vi "UpdateUserInterface.vi"(8 "error in (no error)":errorcluster, 10 "DataExchange":T1, 11 "LaserController in":refnum<class "LaserController.lvclass">) -> (0 "error out":errorcluster, 2 "DataExchange Out":T1, 3 "LaserController out":refnum<class "LaserController.lvclass">)   [LabVIEW 2020, in "LaserController.lvlib" / "LaserController.lvclass"]
uses:
  LaserController.lvclass
  Model/Hardware Abstraction Layer/Component/Device/Device/DataExchange.ctl
  LaserController.lvclass/LaserController.ctl
  Model/Hardware Abstraction Layer/Component/GenericActor/GenericActor/GenericController.lvclass
  Interface/DataListener/DataListener.lvclass
panel:
  in  "event data":cluster{"Label":string, "Value":dbl}
  out "error out 2":errorcluster
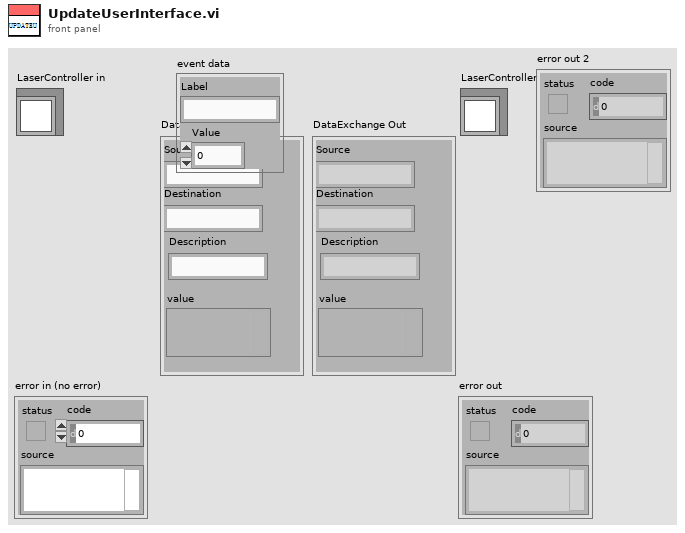
[diagram p1: front panel]
types:
  T1 = typedef "DataListener.lvclass/DataExchange.ctl" = cluster{"Source":string, "Destination":string, "Description":string, "value":variant}
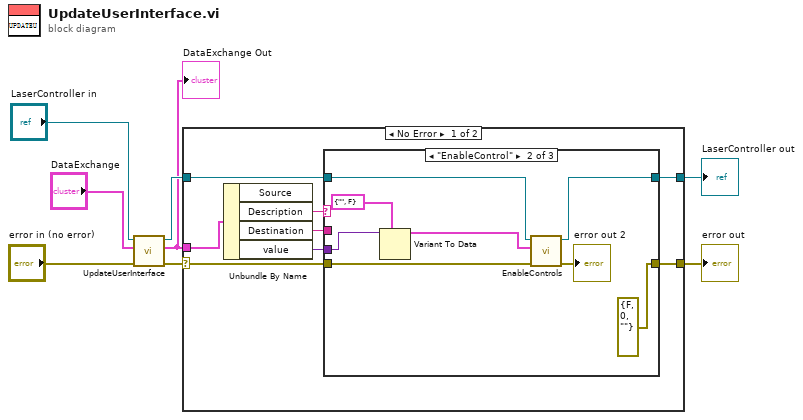
[diagram p0: block diagram]
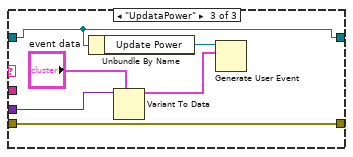
[diagram p3: hidden frame]
diagram:
  n1 = call-parent "UpdateUserInterface.vi"("error in (no error)"="error in (no error)", "DataExchange"="DataExchange", "GenericController in"="LaserController in") -> ("error out"=w4:errorcluster, "DataExchange Out"=w1:T1, "GenericController out"=w5:refnum<class "LaserController.lvclass">)  [unwired: 6 in]
  "DataExchange Out" <- w1
  n2 = case shown="No Error" w4 {
    selector: w4 -> [w10 w34]
    tunnel: [w9 w34] -> w2
    tunnel: [w11 w33] -> w3
    tunnel: w5 -> [w12 w33]
    tunnel: w1 -> [w16 _]
    frame No Error {
      n3 = Unbundle By Name(w16) -> ("Description"=w13:string, "Destination"=w14:string, "value"=w15:variant)  [unwired: 1 out]
      n4 = case shown="\"EnableControl\"" w13 {
        tunnel: w15 -> [_ w26 w32]
        tunnel: w14 -> [_ _ _]
        tunnel: w12 -> [w18 w24 w28]
        tunnel: [w18 w23 w28] -> w11
        tunnel: [w17 errorcluster {"status"=FALSE, "code"=0, "source"=""} ("error IO") w27] -> w9
        tunnel: w10 -> [w17 w25 w27]
        frame "False", Default {
        }
        frame "EnableControl" {
          n5 = Variant To Data(type=cluster{"Label":string, "Visable?":bool} {"Label"="", "Visable?"=FALSE} ("event data"), Variant=w26) -> (data=w19:cluster{"Label":string, "Visable?":bool})  [unwired: 1 in, 1 out]
          n6 = call-dynamic "EnableControls.vi"("error in (no error)"=w25, "event data"=w19, "OxxiusLaserController in"=w24) -> ("error out"=→"error out 2":errorcluster, "OxxiusLaserController out"=w23:refnum<class "LaserController.lvclass">)  [unwired: 7 in]
        }
        frame "UpdataPower" {
          n7 = Unbundle By Name(w28) -> ("Update Power"=w31:refnum<user-event>)
          n8 = Variant To Data(type="event data", Variant=w32) -> (data=w29:cluster{"Label":string, "Value":dbl})  [unwired: 1 in, 1 out]
          n9 = Generate User Event(user event=w31, event data cluster=w29) -> ()  [unwired: 2 in, 2 out]
        }
      }
    }
    frame Error {
    }
  }
  "error out" <- w2
  "LaserController out" <- w3
